vi "Get Waypoint Transfer Status.vi"(8 "Error In":errorcluster) -> (0 "Error Out":errorcluster, 3 "Waypoint Transfer Status Out":T1)   [LabVIEW 2014]
uses:
  Controls/Waypoint Transfer Status.ctl
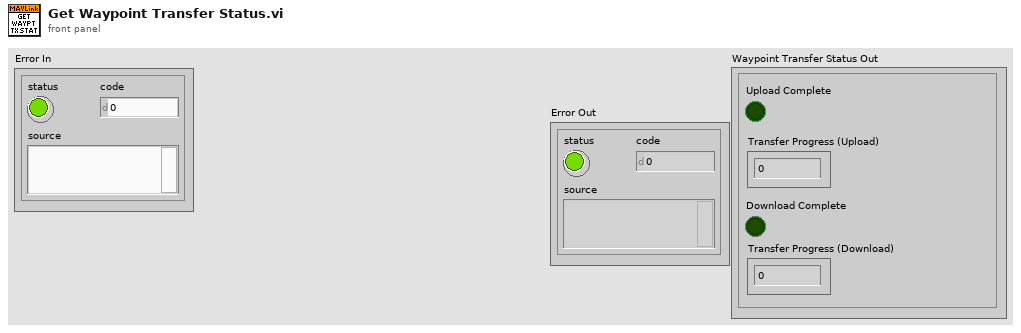
[diagram p1: front panel]
types:
  T1 = typedef "Waypoint Transfer Status.ctl" = cluster{"Upload Complete":bool, "Transfer Progress (Upload)":dbl, "Download Complete":bool, "Transfer Progress (Download)":dbl}
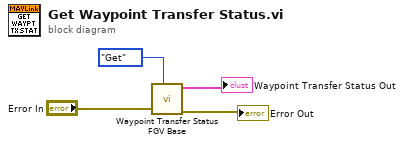
[diagram p0: block diagram]
diagram:
  n1 = call "Waypoint Transfer Status FGV Base.vi"("Method"=enum16{"Get", "Set"}."Get", "Error In"="Error In") -> ("Error Out"=→"Error Out":errorcluster, "Waypoint Type Out"=→"Waypoint Transfer Status Out":T1)  [unwired: 8 in]
